vi "AlicatMFC.vi"(7 "Value to Output":dbl format="%_2f", 8 "Ch Description":T1={"Ch Name"="GRC-A:N2-1:SP(%)", "Type"="AalborgMFC", "Function"=enum."Analogue Output", "Ch State"=enum."On", "Calibration type"="Raw", "A"=0.0, "B"=0.0, "C"=0.0, "D"=0.0, "Comments"="!ASYNC", "Address"={"Main"=170, "Ch."=0, "Sub"=0, "Port Name"="tcp://192.168.126.152:10001/"}, "String"="Front Panel", "Duty"=65535} {"Duty" format="%016b"; "D" format="%#_5g"; "C" format="%#_5g"; "B" format="%#_5g"; "A" format="%#_5g"}) -> (0 "Scan comment":string, 1 "Reading":dbl=nan format="%_3f", 3 "HelpText":string="Analogue Input: Ch0 Mdot; Ch1 Press; Ch2 Temp; Ch3 SP; Ch4 Gas#\nAnalogue Input Ch >10: Reads Ch# register\nAnalogue Output: puts valve in auto, sets setpoint, reads setpoint\nNegative demand will set valve to \"Hold Close\"\nDigital Output: 0-\"Hold Close\", else-Automatic\nCal Constants are stored in  A, B, C, D  of RP(%) channels")   [LabVIEW 2021]
uses:
  ADAM Client/Sub VIs/ADAM Controls/Ch_description_ADAM.ctl
  ADAM Client/Sub VIs/ADAM Controls/Module_type_ADAM.ctl
  ADAM Client/Sub VIs/ADAM Controls/Function_ADAM.ctl
  ADAM Client/Sub VIs/ADAM Controls/Channel_State.ctl
  ADAM Client/Sub VIs/ADAM Controls/Calib_type_ADAM.ctl
  ADAM Client/Sub VIs/ADAM Controls/Address.ctl
  2b84bda5-e46d-a442-a45e-e68b2d2fad50.vi
panel:
  out "tries":i32
  out "execTimeAvg":dbl caption="Avg Execution Time" format="%_3ps"
  out "nCalls":dbl
  out "execTime":dbl caption="Execution Time" format="%_3ps"
  out "GoodComms":bool
  # "VI to control Aalborg Digital Mass Flow Controller"
  # "https://www.aalborg.com/index.php/main_page/product_overview/id_product_overview/24"
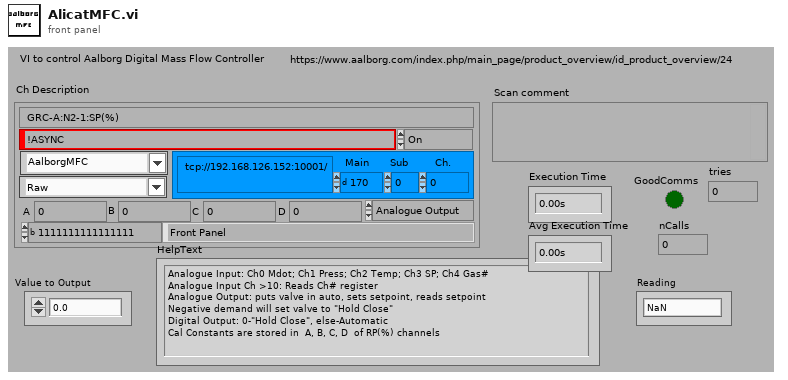
[diagram p1: front panel]
types:
  T1 = typedef "Ch_description_ADAM.ctl" = cluster{"Ch Name":string, "Type":T2, "Function":T3, "Ch State":T4, "Calibration type":T5, "A":dbl, "B":dbl, "C":dbl, "D":dbl, "Comments":string, "Address":T6, "String":string, "Duty":u16}
  T2 = typedef "Module_type_ADAM.ctl" = string
  T3 = typedef "Function_ADAM.ctl" = enum16{"Analogue Input", "Digital Input", "Event counter", "Event rate", "Analogue Output", "Digital Output", "Relay Output"}
  T4 = typedef "Channel_State.ctl" = enum16{"On", "Off", "Always On", "Always Off"}
  T5 = typedef "Calib_type_ADAM.ctl" = string
  T6 = typedef "Address.ctl" = cluster{"Main":i32, "Ch.":i32, "Sub":i32, "Port Name":string}
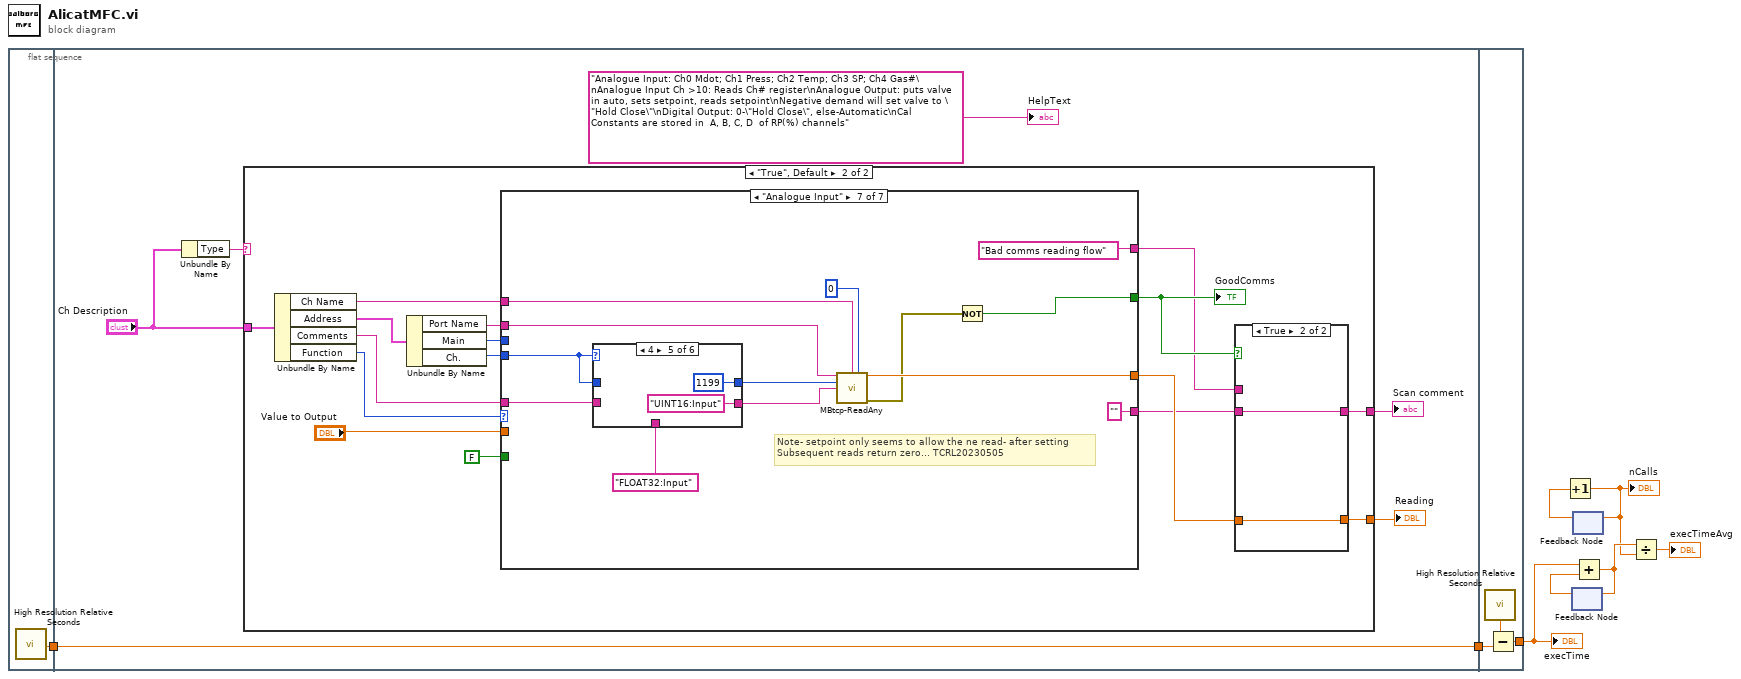
[diagram p0: block diagram]
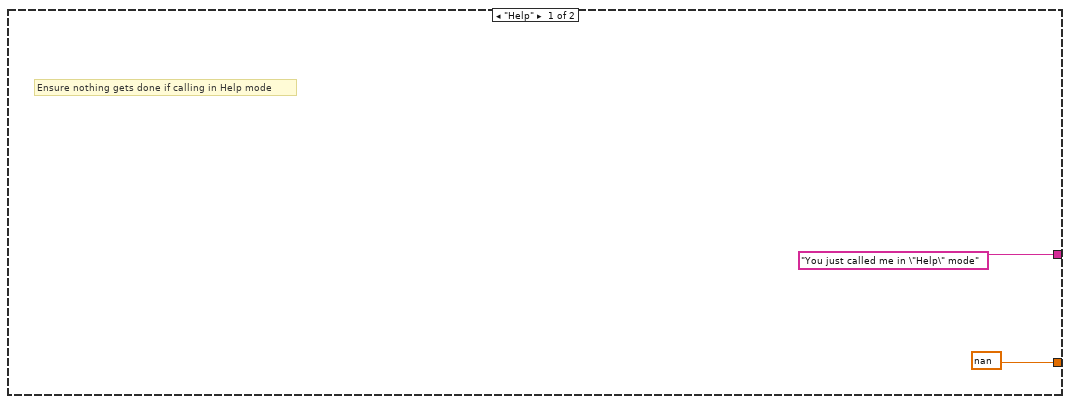
[diagram p2: hidden frame]
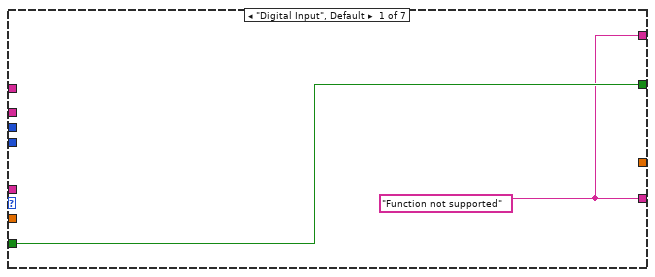
[diagram p3: hidden frame]
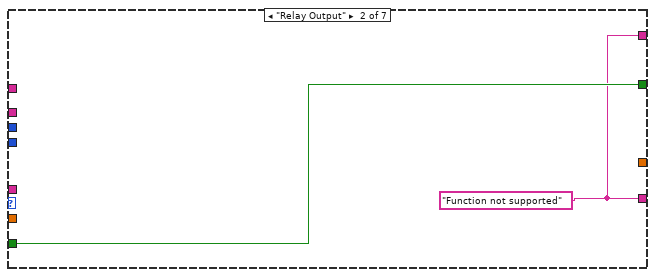
[diagram p4: hidden frame]
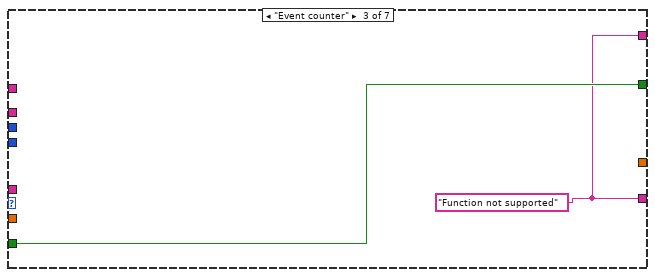
[diagram p5: hidden frame]
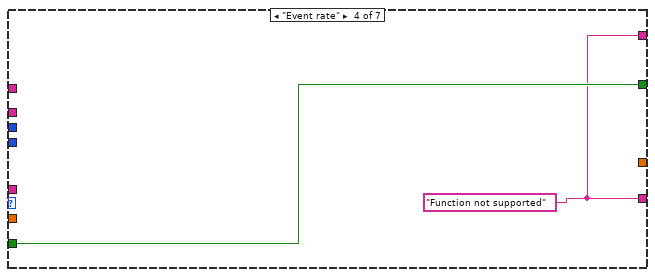
[diagram p6: hidden frame]
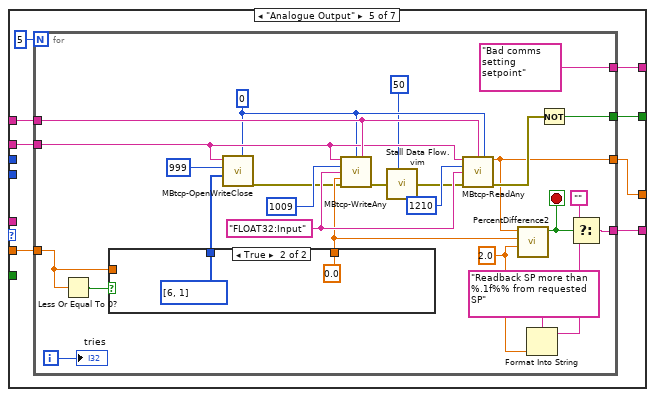
[diagram p7: hidden frame]
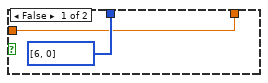
[diagram p8: hidden frame]
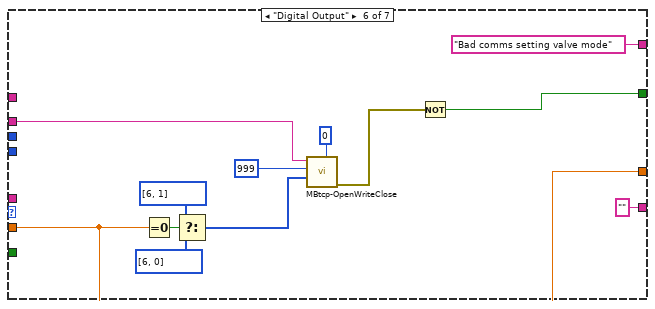
[diagram p9: hidden frame]
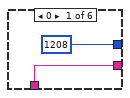
[diagram p10: hidden frame]
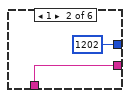
[diagram p11: hidden frame]
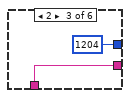
[diagram p12: hidden frame]
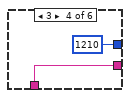
[diagram p13: hidden frame]
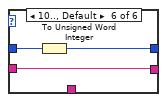
[diagram p14: hidden frame]
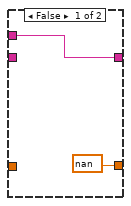
[diagram p15: hidden frame]
diagram:
  n1 = flat-sequence {
    tunnel: [w9] -> w8
    tunnel: w8 -> [w15]
    tunnel: [w15] -> w7
    tunnel: w7 -> [w123]
    tunnel: [w122] -> w1
    frame #0 {
      n2 = call <vilib>:"High Resolution Relative Seconds.vi"() -> ("relative seconds"=w9:dbl)
    }
    frame #1 {
      n3 = Unbundle By Name("Ch Description") -> ("Type"=w12:T2)
      n4 = case shown="\"True\", Default" w12 {
        tunnel: "Ch Description" -> [_ w33]
        tunnel: ["You just called me in \"Help\" mode" w20] -> w13
        tunnel: [nan ("t") w19] -> w14
        frame "Help" {
          # "Ensure nothing gets done if calling in Help mode"
        }
        frame "True", Default {
          n5 = Unbundle By Name(w33) -> ("Ch Name"=w27:string, "Address"=w31:T6, "Comments"=w21:string, "Function"=w22:T3)
          n6 = Unbundle By Name(w31) -> ("Port Name"=w29:string, "Main"=w30:i32, "Ch."=w23:i32)
          n7 = case shown="\"Analogue Input\"" w22 {
            tunnel: w30 -> [_ _ _ _ _ _ _]
            tunnel: w29 -> [_ _ _ _ w48 w89 w102]
            tunnel: [_ _ _ _ w46 w90 w103] -> w28
            tunnel: w27 -> [_ _ _ _ w49 _ w104]
            tunnel: "Value to Output" -> [_ _ _ _ w47 w90 _]
            tunnel: [w35 w37 w39 w41 w43 w82 w97] -> w26
            tunnel: FALSE -> [w35 w37 w39 w41 _ _ _]
            tunnel: [w34 w36 w38 w40 w45 "" ""] -> w24
            tunnel: w23 -> [_ _ _ _ _ _ w100]
            tunnel: w21 -> [_ _ _ _ _ _ w99]
            tunnel: [w34 w36 w38 w40 w44 "Bad comms setting valve mode" "Bad comms reading flow"] -> w18
            frame "Digital Input", Default {
              w34 = "Function not supported"
            }
            frame "Relay Output" {
              w36 = "Function not supported"
            }
            frame "Event counter" {
              w38 = "Function not supported"
            }
            frame "Event rate" {
              w40 = "Function not supported"
            }
            frame "Analogue Output" {
              n8 = for {
                N: 5 -> [_]
                tunnel: w49 -> [w75]
                tunnel: w48 -> [w74]
                tunnel: w47 -> [w64]
                tunnel: [w61] -> w46
                tunnel: [w59] -> w45
                tunnel: ["Bad comms setting setpoint"] -> w44
                tunnel: [w52] -> w43
                i -> [w50]
                stop <- w51 stop-if-true
                w58 = 2.0 ("y")
                w67 = "FLOAT32:Input" ("DataType(:RegisterType)")
                w69 = u8 0 ("Slave ID")
                n9 = Less Or Equal To 0?(x=w64) -> (x <= 0?=w65:bool)
                n10 = case shown="True" w65 {
                  tunnel: [u16[] [6, 0] ("Values") u16[] [6, 1] ("Values")] -> w73
                  tunnel: w64 -> [w76 _]
                  tunnel: [w76 0.0 ("Value to Output")] -> w60
                  frame False {
                  }
                  frame True {
                  }
                }
                n11 = call "MBtcp-OpenWriteClose.vi"("Slave ID"=w69, "Values"=w73, "RegisterAddr"=u16 999, "IP Address(:port)"=w74) -> ("error out"=w53:errorcluster)  [unwired: 7 in]
                n12 = call "MBtcp-WriteAny.vi"("IP Address"=w74, "Slave ID"=w69, "Ch Name"=w75, "Register"=1009, "DataType(:RegisterType)"=w67, "Value to Output"=w60, "Error In"=w53) -> ("error out"=w70:errorcluster)  [unwired: 8 in]
                n13 = call "Stall Data Flow.vim"("value in"=w70, "milliseconds to wait"=u32 50) -> ("value out"=w63:errorcluster)  [unwired: 1 out]
                n14 = call "MBtcp-ReadAny.vi"("IP Address"=w74, "Ch Name"=w75, "Slave ID"=w69, "Register"=u16 1210, "DataType(:RegisterType)"=w67, "Error In"=w63) -> ("Value"=w61:dbl, "error out"=w66:errorcluster)  [unwired: 7 in, 1 out]
                n15 = call "PercentDifference2.vi"("percent+/-"=w58, "target"=w60, "achieved"=w61) -> ("closeEnough"=w51:bool)  [unwired: 7 in, 1 out]
                n16 = Format Into String(format string="Readback SP more than %.1f%% from requested SP", w58) -> (resulting string=w56:string)  [unwired: 2 in, 1 out]
                n17 = Not(x=w66) -> (.not. x?=w52:bool)
                n18 = Select(t="", s=w51, f=w56) -> (s? t:f=w59:string)
                "tries" <- w50
              }
            }
            frame "Digital Output" {
              n19 = Equal To 0?(x=w90) -> (x = 0?=w91:bool)
              n20 = Select(t=u16[] [6, 1] ("Values"), s=w91, f=u16[] [6, 0] ("Values")) -> (s? t:f=w85:u16[])
              n21 = call "MBtcp-OpenWriteClose.vi"("Slave ID"=u8 0, "Values"=w85, "RegisterAddr"=u16 999, "IP Address(:port)"=w89) -> ("error out"=w83:errorcluster)  [unwired: 7 in]
              n22 = Not(x=w83) -> (.not. x?=w82:bool)
            }
            frame "Analogue Input" {
              # "Note- setpoint only seems to allow the ne read- after setting\nSubsequent reads return zero... TCRL20230505"
              n23 = case shown="4" w100 {
                tunnel: [u16 1208 ("Register") u16 1202 ("Ch.") u16 1204 ("Ch.") u16 1210 ("Ch.") u16 1199 ("Ch.") w115] -> w101
                tunnel: w100 -> [_ _ _ _ _ w117]
                tunnel: [w105 w107 w109 w111 "UINT16:Input" ("Comments") w116] -> w94
                tunnel: w99 -> [_ _ _ _ _ w116]
                tunnel: "FLOAT32:Input" ("DataType(:RegisterType)") -> [w105 w107 w109 w111 _ _]
                frame 0 {
                }
                frame 1 {
                }
                frame 2 {
                }
                frame 3 {
                }
                frame 4 {
                }
                frame 10.., Default {
                  n24 = To Unsigned Word Integer(number=w117) -> (unsigned 16bit integer=w115:u16)
                }
              }
              n25 = call "MBtcp-ReadAny.vi"("IP Address"=w102, "Ch Name"=w104, "Slave ID"=u8 0, "Register"=w101, "DataType(:RegisterType)"=w94) -> ("Value"=w103:dbl, "error out"=w98:errorcluster)  [unwired: 8 in, 1 out]
              n26 = Not(x=w98) -> (.not. x?=w97:bool)
            }
          }
          "GoodComms" <- w26
          n27 = case shown="True" w26 {
            tunnel: [w118 w120] -> w20
            tunnel: [nan ("t") w121] -> w19
            tunnel: w28 -> [_ w121]
            tunnel: w24 -> [_ w120]
            tunnel: w18 -> [w118 _]
            frame False {
            }
            frame True {
            }
          }
        }
      }
      "Reading" <- w14
      "Scan comment" <- w13
      "HelpText" <- "Analogue Input: Ch0 Mdot; Ch1 Press; Ch2 Temp; Ch3 SP; Ch4 Gas#\nAnalogue Input Ch >10: Reads Ch# register\nAnalogue Output: puts valve in auto, sets setpoint, reads setpoint\nNegative demand will set valve to \"Hold Close\"\nDigital Output: 0-\"Hold Close\", else-Automatic\nCal Constants are stored in  A, B, C, D  of RP(%) channels"
    }
    frame #2 {
      n28 = call <vilib>:"High Resolution Relative Seconds.vi"() -> ("relative seconds"=w124:dbl)
      n29 = Subtract(x=w124, y=w123) -> (x-y=w122:dbl)
    }
  }
  n30 = feedback #1() -> (w3:dbl)  [unwired: 1 in]
  n31 = feedback #2() -> (w4:dbl)  [unwired: 1 in]
  n32 = Increment(x=w4) -> (x+1=w5:dbl)
  "nCalls" <- w5
  n33 = feedback-in #2(w5) -> ()
  n34 = Add(x=w1, y=w3) -> (x+y=w6:dbl)
  n35 = feedback-in #1(w6) -> ()
  n36 = Divide(x=w6, y=w5) -> (x/y=→"execTimeAvg":dbl)
  "execTime" <- w1
